vi "PackData.vi"(8 "AcqStatusIn":T2, 11 "data in":T3={"channel 0"=[0, 0], "channel 1"=[0, 0], "channel 2"=[0, 0], "channel 3"=[0, 0], "channel 4"=[0, 0], "channel 5"=[0, 0], "channel 6"=[0, 0], "channel 7"=[0, 0]}) -> (0 "AcqStatusOut":T2, 1 "FrameTagDataPack":u64, 2 "GalvoDataPack":u64[](array[numeric]), 3 "PmtDataPack":u64, 5 "GalvoData":T1, 7 "PmtData":cluster{"Pmt1RawData":i16, "Pmt2RawData":i16})   [LabVIEW 2015]
uses:
  Typedefs/AcqStatus.ctl
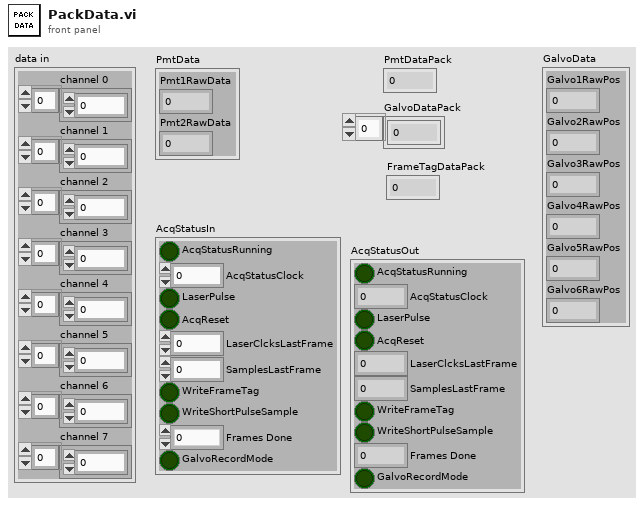
[diagram p1: front panel]
types:
  T1 = cluster{"Galvo1RawPos":i16, "Galvo2RawPos":i16, "Galvo3RawPos":i16, "Galvo4RawPos":i16, "Galvo5RawPos":i16, "Galvo6RawPos":i16}
  T2 = typedef "AcqStatus.ctl" = cluster{"AcqStatusRunning":bool, "AcqStatusClock":u64, "LaserPulse":bool, "AcqReset":bool, "LaserClcksLastFrame":u32, "SamplesLastFrame":u32, "WriteFrameTag":bool, "WriteShortPulseSample":bool, "Frames Done":u32, "GalvoRecordMode":bool}
  T3 = cluster{"channel 0":i16[], "channel 1":i16[], "channel 2":i16[], "channel 3":i16[], "channel 4":i16[], "channel 5":i16[], "channel 6":i16[], "channel 7":i16[]}
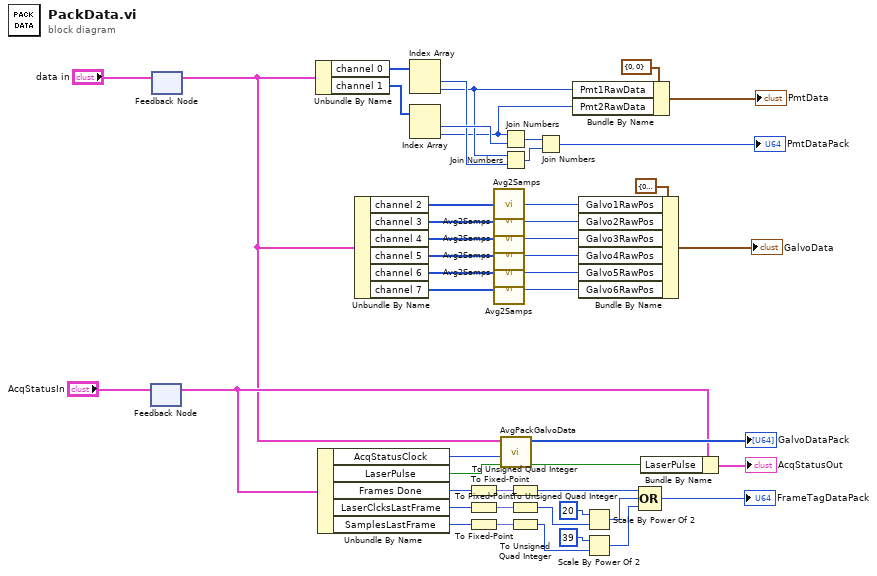
[diagram p0: block diagram]
diagram:
  n1 = feedback-in #1("AcqStatusIn") -> ()
  n2 = feedback #1() -> (w3:T2)  [unwired: 1 in]
  n3 = feedback #2() -> (w1:T3)  [unwired: 1 in]
  n4 = feedback-in #2("data in") -> ()
  n5 = Unbundle By Name(w1) -> ("channel 0"=w43:i16[], "channel 1"=w44:i16[])
  n6 = Unbundle By Name(w3) -> ("AcqStatusClock"=w5:u64, "LaserPulse"=w19:bool, "Frames Done"=w21:u32, "LaserClcksLastFrame"=w36:u32, "SamplesLastFrame"=w35:u32)
  n7 = Unbundle By Name(w1) -> ("channel 2"=w23:i16[], "channel 3"=w16:i16[], "channel 4"=w14:i16[], "channel 5"=w12:i16[], "channel 6"=w10:i16[], "channel 7"=w8:i16[])
  n8 = Index Array(array=w43) -> (element #1=w41:i16, element #2=w40:i16)  [unwired: 2 in]
  n9 = Index Array(array=w44) -> (element #1=w42:i16, element #2=w39:i16)  [unwired: 2 in]
  n10 = To Fixed-Point(number=w21) -> (fixed-point=w34:fxp<+,20,20>)  [unwired: 1 in]
  n11 = To Fixed-Point(number=w36) -> (fixed-point=w33:fxp<+,19,19>)  [unwired: 1 in]
  n12 = To Fixed-Point(number=w35) -> (fixed-point=w32:fxp<+,25,25>)  [unwired: 1 in]
  n13 = call "Avg2Samps.vi"("channel in"=w23) -> ("Numeric"=w22:i16)  [unwired: 4 in]
  n14 = call "Avg2Samps.vi"("channel in"=w16) -> ("Numeric"=w15:i16)  [unwired: 4 in]
  n15 = call "Avg2Samps.vi"("channel in"=w14) -> ("Numeric"=w13:i16)  [unwired: 4 in]
  n16 = call "Avg2Samps.vi"("channel in"=w12) -> ("Numeric"=w11:i16)  [unwired: 4 in]
  n17 = call "Avg2Samps.vi"("channel in"=w10) -> ("Numeric"=w9:i16)  [unwired: 4 in]
  n18 = call "Avg2Samps.vi"("channel in"=w8) -> ("Numeric"=w7:i16)  [unwired: 4 in]
  n19 = Join Numbers(hi=w39, lo=w42) -> ((hi.lo)=w45:u32)
  n20 = Join Numbers(hi=w40, lo=w41) -> ((hi.lo)=w46:u32)
  n21 = call "AvgPackGalvoData.vi"("Laser Pulse"=w19, "AcqStatusClock"=w5, "data in"=w1) -> ("Data Valid Out"=w6:bool, "GalvoDataPack"=→"GalvoDataPack":u64[])  [unwired: 7 in]
  n22 = To Unsigned Quad Integer(1:w34) -> (0:w29:u64)
  n23 = To Unsigned Quad Integer(1:w33) -> (0:w31:u64)
  n24 = To Unsigned Quad Integer(1:w32) -> (0:w30:u64)
  n25 = Join Numbers(hi=w45, lo=w46) -> ((hi.lo)=→"PmtDataPack":u64)
  n26 = Bundle By Name(cluster=cluster{"Pmt1RawData":i16, "Pmt2RawData":i16} {"Pmt1RawData"=0, "Pmt2RawData"=0}, "Pmt1RawData"=w40, "Pmt2RawData"=w39) -> (→"PmtData":cluster{"Pmt1RawData":i16, "Pmt2RawData":i16})
  n27 = Bundle By Name(cluster=T1 {"Galvo1RawPos"=0, "Galvo2RawPos"=0, "Galvo3RawPos"=0, "Galvo4RawPos"=0, "Galvo5RawPos"=0, "Galvo6RawPos"=0}, "Galvo1RawPos"=w22, "Galvo2RawPos"=w15, "Galvo3RawPos"=w13, "Galvo4RawPos"=w11, "Galvo5RawPos"=w9, "Galvo6RawPos"=w7) -> (→"GalvoData":T1)
  n28 = Scale By Power Of 2(n=i16 20, x=w31) -> (x*2^n=w28:u64)
  n29 = Scale By Power Of 2(n=i16 39, x=w30) -> (x*2^n=w27:u64)
  n30 = Compound Arithmetic op=OR(w29, w28, w27) -> (→"FrameTagDataPack":u64)
  n31 = Bundle By Name(cluster=w3, "LaserPulse"=w6) -> (→"AcqStatusOut":T2)
